vi "GetControlValueByPathString.vi"(0 "VI Reference In":refnum<vi>, 2 "delimiter (>>)":string=">>", 5 "Control Name":string, 11 "error in":errorcluster) -> (4 "VI Reference Out":refnum<vi>, 6 "Value":variant, 15 "error out":errorcluster)   [LabVIEW 2016, in "Drona.lvlib" / "GetControlValue.lvlib"]
doc: "Gives the value of controls. \nThe input control name is given as a string , incase of path, use delimiters inbetween the path."
uses:
  GetControlValue.lvlib
  Drona.lvlib
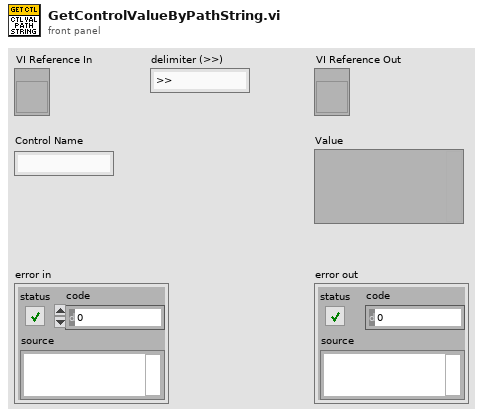
[diagram p1: front panel]
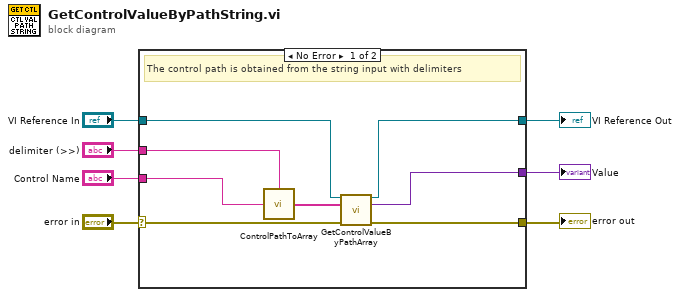
[diagram p0: block diagram]
diagram:
  n1 = case shown="No Error" "error in" {
    selector: "error in" -> [w14 w17]
    tunnel: "Control Name" -> [w9 _]
    tunnel: "VI Reference In" -> [w15 w16]
    tunnel: [w12 w16] -> w4
    tunnel: [w13 w17] -> w3
    tunnel: [w11 _] -> w2
    tunnel: "delimiter (>>)" -> [w8 _]
    frame No Error {
      # "The control path is obtained from the string input with delimiters"
      n2 = call "ControlPathToArray.vi"("Control Name"=w9, "delimiter (>>)"=w8) -> ("Control Path"=w10:string[])
      n3 = call "GetControlValueByPathArray.vi"("VI Reference In"=w15, "Control Path"=w10, "error in"=w14) -> ("VI Reference Out"=w12:refnum<vi>, "Value"=w11:variant, "error out"=w13:errorcluster)  [unwired: 10 in]
    }
    frame Error {
    }
  }
  "error out" <- w3
  "VI Reference Out" <- w4
  "Value" <- w2
